vi "Write Type.vi"(8 "error in (no error)":errorcluster, 10 "Module type":T1, 11 "Library in":refnum<class "Library.lvclass">) -> (0 "error out":errorcluster, 3 "Library out":refnum<class "Library.lvclass">)   [LabVIEW 2019, in "Panther Dashboard.lvlib" / "Library.lvclass"]
uses:
  Library.lvclass
  Panther Dashboard/Module type--enum.ctl
  Library.lvclass/Library.ctl
  Panther Dashboard/Panther Dashboard.lvlib
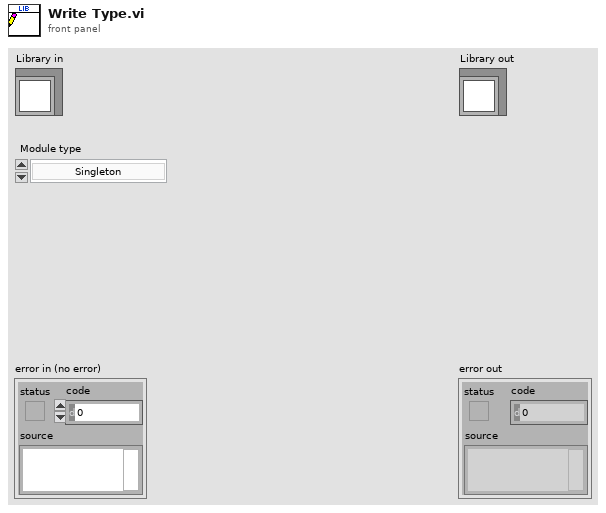
[diagram p1: front panel]
types:
  T1 = typedef "Panther Dashboard.lvlib/Module type--enum.ctl" = enum16{"Singleton", "Cloneable"}
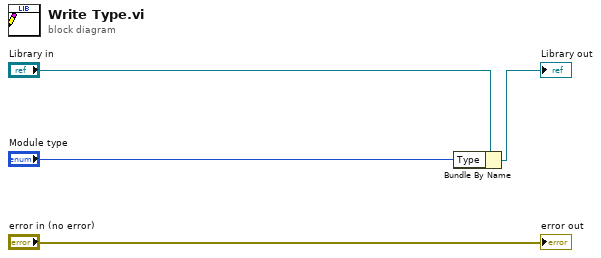
[diagram p0: block diagram]
diagram:
  n1 = Bundle By Name(cluster="Library in", "Type"="Module type") -> (→"Library out":refnum<class "Library.lvclass">)
  "error out" <- "error in (no error)"
